vi "Get Common Type.vi"(11 "JSON Array":refnum<class "JSON Array.lvclass">) -> ()   [LabVIEW 2017, in "JSON Array.lvclass"]
uses:
  JSON Array.lvclass
  JSON Types.ctl
  JSON Array.lvclass/JSON Array.ctl
  JSON Datatype/JSON Datatype.lvclass
panel:
  out "Array":T1[](array[typedef])
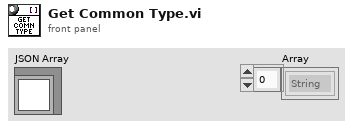
[diagram p1: front panel]
types:
  T1 = typedef "JSON Types.ctl" = enum16{"String", "Numeric", "Boolean", "NULL", "Object", "1D Array", "1D String", "1D Numeric", "1D Boolean"}
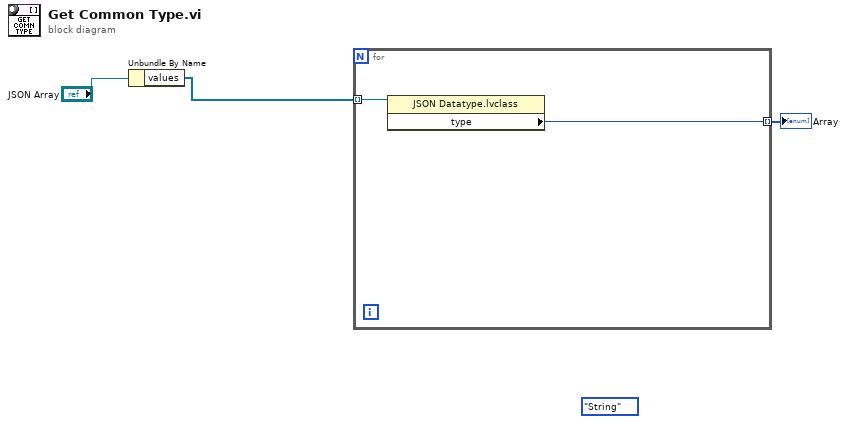
[diagram p0: block diagram]
diagram:
  (unwired) JSON_Types."String" ("type")
  n1 = Unbundle By Name("JSON Array") -> ("values"=w2:refnum<class "JSON Datatype.lvclass">[])
  n2 = for {
    tunnel: w2 -> [w5] mode=indexing
    tunnel: [w4] -> w1 mode=indexing
    n3 = property class="JSON Datatype.lvclass"(reference=w5) -> ("type"=w4:T1)  [unwired: 1 in, 2 out]
  }
  "Array" <- w1
